vi "SMS Candidate Selection.vi"(0 "Image Ref (U16)":T1, 7 "Blink Sensitivity":sgl=1.3, 11 "Error In":errorcluster) -> (4 "Image Ref (U16) - Dup":T1, 8 "Cadidate Image Ref":T1, 15 "Error Out":errorcluster)   [LabVIEW 2020]
uses:
  <vilib>/vision/Image Controls.llb/IMAQ Image.ctl
  <vilib>/vision/NI_Vision_Development_Module.lvlib
panel:
  out "Image border size out":i32
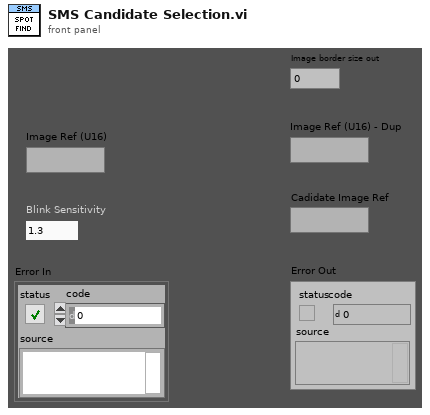
[diagram p1: front panel]
types:
  T1 = typedef "IMAQ Image.ctl" = refnum<image>
  T2 = typedef "Image Type" = u32
  T3 = enum32{"Average", "Min", "Max", "Clear  if < ", "Clear  if < or =", "Clear  if =", "Clear  if > or =", "Clear  if >"}
  T4 = enum32{"AutoM", "Close", "Dilate", "Erode", "Gradient", "Gradient in", "Gradient out", "HitMiss", "Open", "PClose", "POpen", "Thick", "Thin"}
  T5 = cluster{"histogram":u32[], "Minimal Value":sgl, "Maximal Value":sgl, "Starting Value":sgl, "Interval Width":sgl, "Mean Value":sgl, "Standard  Variation":sgl, "Area (pixels)":i32}
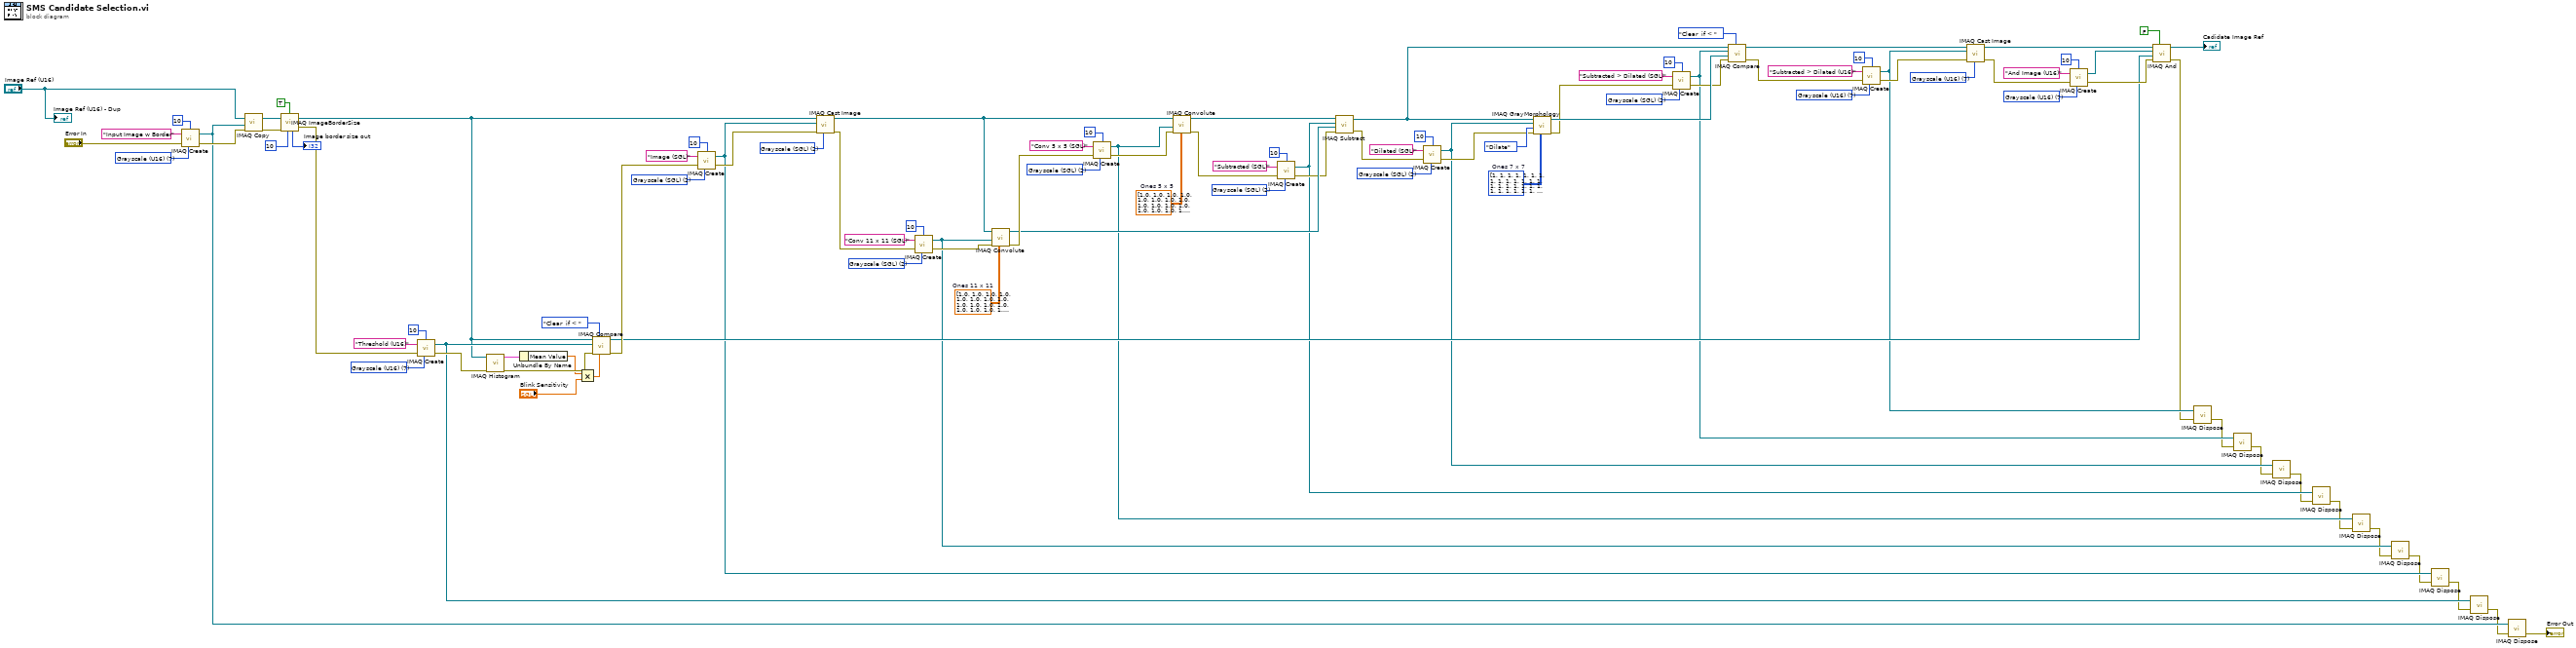
[diagram p0: block diagram]
diagram:
  w16 = T2 7 items=["Grayscale (U8)", "Grayscale (I16)", "Grayscale (SGL)", "Complex (CSG)", "RGB (U32)", "HSL (U32)", "RGB (U64)", "Grayscale (U16)"] ("Image Type")
  w39 = T2 7 items=["Grayscale (U8)", "Grayscale (I16)", "Grayscale (SGL)", "Complex (CSG)", "RGB (U32)", "HSL (U32)", "RGB (U64)", "Grayscale (U16)"] ("Image Type")
  w49 = T2 7 items=["Grayscale (U8)", "Grayscale (I16)", "Grayscale (SGL)", "Complex (CSG)", "RGB (U32)", "HSL (U32)", "RGB (U64)", "Grayscale (U16)"] ("Image Type")
  w51 = T2 7 items=["Grayscale (U8)", "Grayscale (I16)", "Grayscale (SGL)", "Complex (CSG)", "RGB (U32)", "HSL (U32)", "RGB (U64)", "Grayscale (U16)"] ("Image Type")
  w54 = T2 2 items=["Grayscale (U8)", "Grayscale (I16)", "Grayscale (SGL)", "Complex (CSG)", "RGB (U32)", "HSL (U32)", "RGB (U64)", "Grayscale (U16)"] ("Image Type")
  w60 = i32[][] [[1, 1, 1, 1, 1, 1, 1], [1, 1, 1, 1, 1, 1, 1], [1, 1, 1, 1, 1, 1, 1], [1, 1, 1, 1, 1, 1, 1], [1, 1, 1, 1, 1, 1, 1], [1, 1, 1, 1, 1, 1, 1], [1, 1, 1, 1, 1, 1, 1]]  # Ones 7 x 7
  w64 = T2 2 items=["Grayscale (U8)", "Grayscale (I16)", "Grayscale (SGL)", "Complex (CSG)", "RGB (U32)", "HSL (U32)", "RGB (U64)", "Grayscale (U16)"] ("Image Type")
  w73 = T2 2 items=["Grayscale (U8)", "Grayscale (I16)", "Grayscale (SGL)", "Complex (CSG)", "RGB (U32)", "HSL (U32)", "RGB (U64)", "Grayscale (U16)"] ("Image Type")
  w80 = T2 7 items=["Grayscale (U8)", "Grayscale (I16)", "Grayscale (SGL)", "Complex (CSG)", "RGB (U32)", "HSL (U32)", "RGB (U64)", "Grayscale (U16)"] ("Image Type")
  w90 = T2 2 items=["Grayscale (U8)", "Grayscale (I16)", "Grayscale (SGL)", "Complex (CSG)", "RGB (U32)", "HSL (U32)", "RGB (U64)", "Grayscale (U16)"] ("Image Type")
  w91 = T2 2 items=["Grayscale (U8)", "Grayscale (I16)", "Grayscale (SGL)", "Complex (CSG)", "RGB (U32)", "HSL (U32)", "RGB (U64)", "Grayscale (U16)"] ("Image Type")
  w94 = sgl[][] [[1.0, 1.0, 1.0, 1.0, 1.0, 1.0, 1.0, 1.0, 1.0, 1.0, 1.0], [1.0, 1.0, 1.0, 1.0, 1.0, 1.0, 1.0, 1.0, 1.0, 1.0, 1.0], [1.0, 1.0, 1.0, 1.0, 1.0, 1.0, 1.0, 1.0, 1.0, 1.0, 1.0], [1.0, 1.0, 1.0, 1.0, 1.0, 1.0, 1.0, 1.0, 1.0, 1.0, 1.0], [1.0, 1.0, 1.0, 1.0, 1.0, 1.0, 1.0, 1.0, 1.0, 1.0, 1.0], [1.0, 1.0, 1.0, 1.0, 1.0, 1.0, 1.0, 1.0, 1.0, 1.0, 1.0], [1.0, 1.0, 1.0, 1.0, 1.0, 1.0, 1.0, 1.0, 1.0, 1.0, 1.0], [1.0, 1.0, 1.0, 1.0, 1.0, 1.0, 1.0, 1.0, 1.0, 1.0, 1.0], [1.0, 1.0, 1.0, 1.0, 1.0, 1.0, 1.0, 1.0, 1.0, 1.0, 1.0], [1.0, 1.0, 1.0, 1.0, 1.0, 1.0, 1.0, 1.0, 1.0, 1.0, 1.0], [1.0, 1.0, 1.0, 1.0, 1.0, 1.0, 1.0, 1.0, 1.0, 1.0, 1.0]]  # Ones 11 x 11
  w95 = sgl[][] [[1.0, 1.0, 1.0, 1.0, 1.0], [1.0, 1.0, 1.0, 1.0, 1.0], [1.0, 1.0, 1.0, 1.0, 1.0], [1.0, 1.0, 1.0, 1.0, 1.0], [1.0, 1.0, 1.0, 1.0, 1.0]]  # Ones 5 x 5
  w99 = T2 2 items=["Grayscale (U8)", "Grayscale (I16)", "Grayscale (SGL)", "Complex (CSG)", "RGB (U32)", "HSL (U32)", "RGB (U64)", "Grayscale (U16)"] ("Image Type")
  w100 = T2 2 items=["Grayscale (U8)", "Grayscale (I16)", "Grayscale (SGL)", "Complex (CSG)", "RGB (U32)", "HSL (U32)", "RGB (U64)", "Grayscale (U16)"] ("Image Type")
  n1 = call "IMAQ Create"("Border Size"=10, "Image Name"="Input Image w Border", "Image Type"=w16, "error in (no error)"="Error In") -> ("New Image"=w11:T1, "error out"=w13:errorcluster)  [unwired: 1 in]
  n2 = call "IMAQ Copy"("error in (no error)"=w13, "Image Dst"=w11, "Image Src"="Image Ref (U16)") -> ("error out"=w4:errorcluster, "Image Dst Out"=w8:T1)  [unwired: 3 in]
  n3 = call "IMAQ ImageBorderSize"("Get/Set Status? (Set)"=TRUE, "Image"=w8, "Image border size in"=10, "error in (no error)"=w4) -> ("Image Out"=w6:T1, "error out"=w3:errorcluster, "Image border size out"=→"Image border size out":i32)
  n4 = call "IMAQ Create"("Border Size"=10, "Image Name"="Threshold (U16)", "Image Type"=w80, "error in (no error)"=w3) -> ("New Image"=w33:T1, "error out"=w41:errorcluster)  [unwired: 1 in]
  n5 = call "IMAQ Histogram"("error in (no error)"=w41, "Image"=w6) -> ("error out"=w79:errorcluster, "Histogram Report"=w76:T5)  [unwired: 8 in]
  n6 = Unbundle By Name(w76) -> ("Mean Value"=w75:sgl)
  n7 = Multiply(x=w75, y="Blink Sensitivity") -> (x*y=w74:sgl)
  n8 = call "IMAQ Compare"("Constant"=w74, "Operator"=T3."Clear  if < ", "error in (no error)"=w79, "Image Dst"=w33, "Image Src A"=w6) -> ("error out"=w42:errorcluster, "Image Dst Out"=w35:T1)  [unwired: 5 in]
  n9 = call "IMAQ Create"("Border Size"=10, "Image Name"="Image (SGL)", "Image Type"=w99, "error in (no error)"=w42) -> ("New Image"=w32:T1, "error out"=w84:errorcluster)  [unwired: 1 in]
  n10 = call "IMAQ Cast Image"("Image Type"=w100, "error in (no error)"=w84, "Image Dst"=w32, "Image Src"=w6) -> ("error out"=w83:errorcluster, "Image Dst Out"=w96:T1)  [unwired: 6 in]
  n11 = call "IMAQ Create"("Border Size"=10, "Image Name"="Conv 11 x 11 (SGL)", "Image Type"=w90, "error in (no error)"=w83) -> ("New Image"=w31:T1, "error out"=w87:errorcluster)  [unwired: 1 in]
  n12 = call "IMAQ Convolute"("Kernel"=w94, "error in (no error)"=w87, "Image Dst"=w31, "Image Src"=w96) -> ("error out"=w85:errorcluster, "Image Dst Out"=w69:T1)  [unwired: 6 in]
  n13 = call "IMAQ Create"("Border Size"=10, "Image Name"="Conv 5 x 5 (SGL)", "Image Type"=w91, "error in (no error)"=w85) -> ("New Image"=w30:T1, "error out"=w86:errorcluster)  [unwired: 1 in]
  n14 = call "IMAQ Convolute"("Kernel"=w95, "error in (no error)"=w86, "Image Dst"=w30, "Image Src"=w96) -> ("error out"=w68:errorcluster, "Image Dst Out"=w70:T1)  [unwired: 6 in]
  n15 = call "IMAQ Create"("Border Size"=10, "Image Name"="Subtracted (SGL)", "Image Type"=w73, "error in (no error)"=w68) -> ("New Image"=w29:T1, "error out"=w67:errorcluster)  [unwired: 1 in]
  n16 = call "IMAQ Subtract"("Image Src A"=w70, "Image Dst"=w29, "Image Src B"=w69, "error in (no error)"=w67) -> ("Image Dst Out"=w58:T1, "error out"=w62:errorcluster)  [unwired: 3 in]
  n17 = call "IMAQ Create"("Border Size"=10, "Image Name"="Dilated (SGL)", "Image Type"=w64, "error in (no error)"=w62) -> ("New Image"=w28:T1, "error out"=w61:errorcluster)  [unwired: 1 in]
  n18 = call "IMAQ GrayMorphology"("Structuring Element"=w60, "error in (no error)"=w61, "Operation"=T4."Dilate", "Image Dst"=w28, "Image Src"=w58) -> ("error out"=w53:errorcluster, "Image Dst Out"=w57:T1)  [unwired: 5 in]
  n19 = call "IMAQ Create"("Border Size"=10, "Image Name"="Subtracted > Dilated (SGL)", "Image Type"=w54, "error in (no error)"=w53) -> ("New Image"=w27:T1, "error out"=w52:errorcluster)  [unwired: 1 in]
  n20 = call "IMAQ Compare"("Operator"=T3."Clear  if < ", "error in (no error)"=w52, "Image Src B"=w57, "Image Dst"=w27, "Image Src A"=w58) -> ("error out"=w46:errorcluster, "Image Dst Out"=w50:T1)  [unwired: 5 in]
  n21 = call "IMAQ Create"("Border Size"=10, "Image Name"="Subtracted > Dilated (U16)", "Image Type"=w49, "error in (no error)"=w46) -> ("New Image"=w26:T1, "error out"=w45:errorcluster)  [unwired: 1 in]
  n22 = call "IMAQ Cast Image"("Image Type"=w51, "error in (no error)"=w45, "Image Dst"=w26, "Image Src"=w50) -> ("error out"=w37:errorcluster, "Image Dst Out"=w43:T1)  [unwired: 6 in]
  n23 = call "IMAQ Create"("Border Size"=10, "Image Name"="And Image (U16)", "Image Type"=w39, "error in (no error)"=w37) -> ("New Image"=w34:T1, "error out"=w36:errorcluster)  [unwired: 1 in]
  n24 = call "IMAQ And"("And/Nand (And)"=FALSE, "error in (no error)"=w36, "Image Src B"=w35, "Image Dst"=w34, "Image Src A"=w43) -> ("error out"=w17:errorcluster, "Image Dst Out"=→"Cadidate Image Ref":T1)  [unwired: 5 in]
  n25 = call "IMAQ Dispose"("Image"=w26, "error in (no error)"=w17) -> ("error out"=w25:errorcluster)  [unwired: 4 in]
  n26 = call "IMAQ Dispose"("Image"=w27, "error in (no error)"=w25) -> ("error out"=w24:errorcluster)  [unwired: 4 in]
  n27 = call "IMAQ Dispose"("Image"=w28, "error in (no error)"=w24) -> ("error out"=w23:errorcluster)  [unwired: 4 in]
  n28 = call "IMAQ Dispose"("Image"=w29, "error in (no error)"=w23) -> ("error out"=w22:errorcluster)  [unwired: 4 in]
  n29 = call "IMAQ Dispose"("Image"=w30, "error in (no error)"=w22) -> ("error out"=w21:errorcluster)  [unwired: 4 in]
  n30 = call "IMAQ Dispose"("Image"=w31, "error in (no error)"=w21) -> ("error out"=w20:errorcluster)  [unwired: 4 in]
  n31 = call "IMAQ Dispose"("Image"=w32, "error in (no error)"=w20) -> ("error out"=w19:errorcluster)  [unwired: 4 in]
  n32 = call "IMAQ Dispose"("Image"=w33, "error in (no error)"=w19) -> ("error out"=w10:errorcluster)  [unwired: 4 in]
  n33 = call "IMAQ Dispose"("Image"=w11, "error in (no error)"=w10) -> ("error out"=→"Error Out":errorcluster)  [unwired: 4 in]
  "Image Ref (U16) - Dup" <- "Image Ref (U16)"
